vi "Create Channels.vi"(8 "error in (no error)":errorcluster, 10 "RSI Module in":refnum<class "RSI Module.lvclass">, 11 "Parent Ref in":T1 format="%.0x") -> (0 "error out":errorcluster, 2 "RSI Module out":refnum<class "RSI Module.lvclass">, 3 "Parent Ref out":T1 format="%.0x")   [LabVIEW 2011, in "Modules.lvlib" / "RSI Module.lvclass"]
uses:
  RSI Module.lvclass
  <vilib>/NI Veristand/Custom Device API/Custom Device Item Ref.ctl
  <vilib>/NI Veristand/Custom Device API/Custom Device Channel Type.ctl
  RSI Module.lvclass/RSI Module.ctl
  <vilib>/NI Veristand/Custom Device API/Custom Device Channel.ctl
  Channel GUIDs.vi
  Class Property Strings.vi
  <vilib>/NI Veristand/Custom Device API/Custom Device API.lvlib
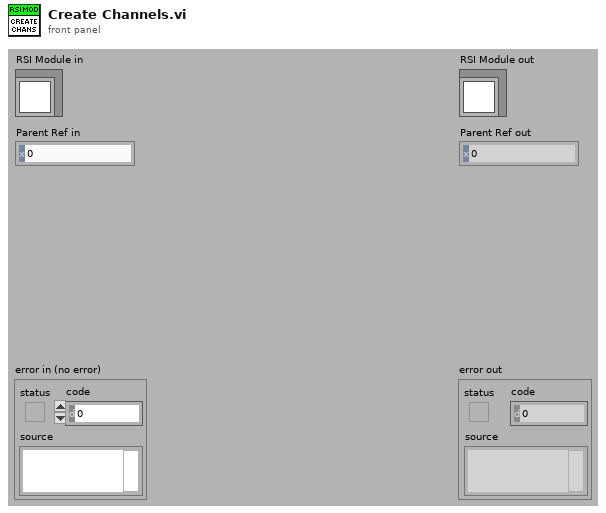
[diagram p1: front panel]
types:
  T1 = typedef "Custom Device API.lvlib/Custom Device Item Ref.ctl" = u64
  T2 = typedef "Custom Device API.lvlib/Custom Device Channel Type.ctl" = enum16{"Input", "Output"}
  T3 = typedef "Custom Device API.lvlib/Custom Device Channel.ctl" = cluster{"Type":T2, "Units":string, "Default Value":dbl, "Faultable":bool, "Scalable":bool}
  T4 = typedef "Modules.lvlib/RSI Module.lvclass/Channel Type.ctl" = enum16{"Analog", "Digital"}
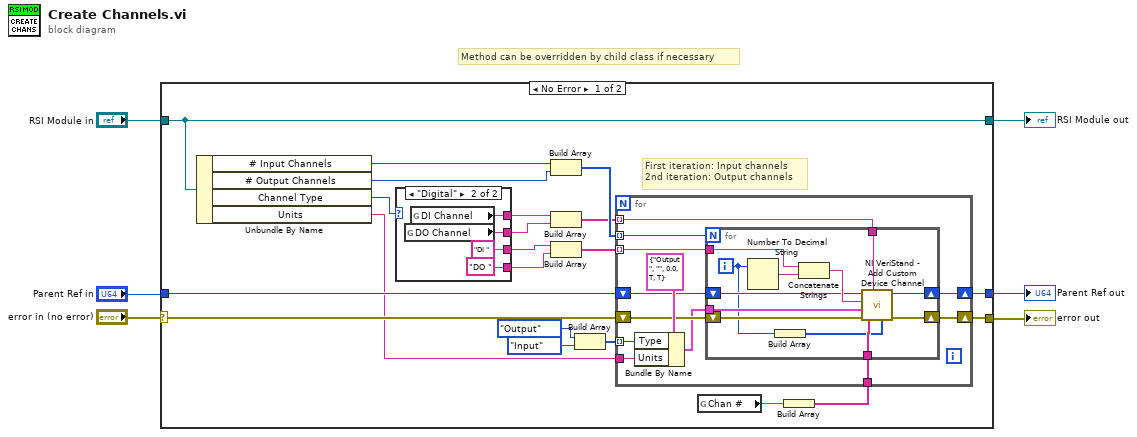
[diagram p0: block diagram]
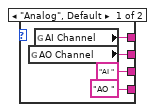
[diagram p2: hidden frame]
diagram:
  # "Method can be overridden by child class if necessary"
  n1 = case shown="No Error" "error in (no error)" {
    selector: "error in (no error)" -> [w14 w62]
    tunnel: [w10 w62] -> w5
    tunnel: [w27 w61] -> w3
    tunnel: "RSI Module in" -> [w27 w61]
    tunnel: "Parent Ref in" -> [w13 w60]
    tunnel: [w9 w60] -> w1
    frame No Error {
      # "First iteration: Input channels\n2nd iteration: Output channels"
      n2 = Unbundle By Name(w27) -> ("# Input Channels"=w26:i32, "# Output Channels"=w25:i32, "Channel Type"=w8:T4, "Units"=w7:string)
      n3 = case shown="\"Digital\"" w8 {
        tunnel: [w55 w59] -> w24
        tunnel: ["AI " ("Channel Name") "DI " ("Channel Name")] -> w22
        tunnel: [w53 w57] -> w23
        tunnel: ["AO " ("Channel Name") "DO " ("Channel Name")] -> w21
        frame "Analog", Default {
          n4 = global read "Channel GUIDs.vi" "AO Channel"() -> (w53:string)
          n5 = global read "Channel GUIDs.vi" "AI Channel"() -> (w55:string)
        }
        frame "Digital" {
          n6 = global read "Channel GUIDs.vi" "DO Channel"() -> (w57:string)
          n7 = global read "Channel GUIDs.vi" "DI Channel"() -> (w59:string)
        }
      }
      n8 = Build Array(w26, w25) -> (w18:i32[])
      n9 = Build Array(w24, w23) -> (w17:string[])
      n10 = Build Array(w22, w21) -> (w16:string[])
      n11 = Build Array(Custom_Device_Channel_Type."Output" ("Type"), Custom_Device_Channel_Type."Input" ("Type")) -> (w15:T2[])
      n12 = global read "Class Property Strings.vi" "Chan #"() -> (w12:string)
      n13 = Build Array(w12) -> (w11:string[])
      n14 = for {
        tunnel: w18 -> [w29] mode=indexing
        tunnel: w17 -> [w33] mode=indexing
        tunnel: w16 -> [w36] mode=indexing
        tunnel: w15 -> [w38] mode=indexing
        tunnel: w11 -> [w32]
        shift-right: [w31] -> w10
        shift-left: w14 -> [w37]
        shift-right: [w30] -> w9
        shift-left: w13 -> [w35]
        tunnel: w7 -> [w28]
        n15 = Bundle By Name(cluster=T3 {"Type"=enum."Output", "Units"="", "Default Value"=0.0, "Faultable"=TRUE, "Scalable"=TRUE} ("Channel"), "Type"=w38, "Units"=w28) -> (w34:T3)
        n16 = for {
          N: w29 -> [_]
          tunnel: w36 -> [w49]
          tunnel: w34 -> [w46]
          tunnel: w33 -> [w45]
          tunnel: w32 -> [w44]
          shift-right: [w41] -> w31
          shift-left: w37 -> [w50]
          shift-right: [w40] -> w30
          shift-left: w35 -> [w47]
          i -> [w43]
          n17 = Number To Decimal String(number=w43) -> (decimal integer string=w51:string)  [unwired: 1 in]
          n18 = Build Array(w43) -> (w42:i32[])
          n19 = Concatenate Strings(w49, w51) -> (w48:string)
          n20 = call <vilib>:"NI VeriStand - Add Custom Device Channel.vi"("Property Values"=w42, "Property names"=w44, "GUID (Default Channel)"=w45, "error in (no error)"=w50, "Channel"=w46, "Channel Name"=w48, "Parent Ref in"=w47) -> ("error out"=w41:errorcluster, "Parent Ref out"=w40:T1)  [unwired: 1 in, 2 out]
        }
      }
    }
    frame Error {
    }
  }
  "error out" <- w5
  "RSI Module out" <- w3
  "Parent Ref out" <- w1
